vi "SetupProcess.vi"(8 "error in (no error)":errorcluster, 10 "SetupData":string, 11 "ScopeBB in":refnum<class "ScopeBB.lvclass">) -> (0 "error out":errorcluster, 2 "Type":string, 3 "ScopeBB out":refnum<class "ScopeBB.lvclass">)   [LabVIEW 2018, in "ScopeBB.lvclass"]
uses:
  ScopeBB.lvclass
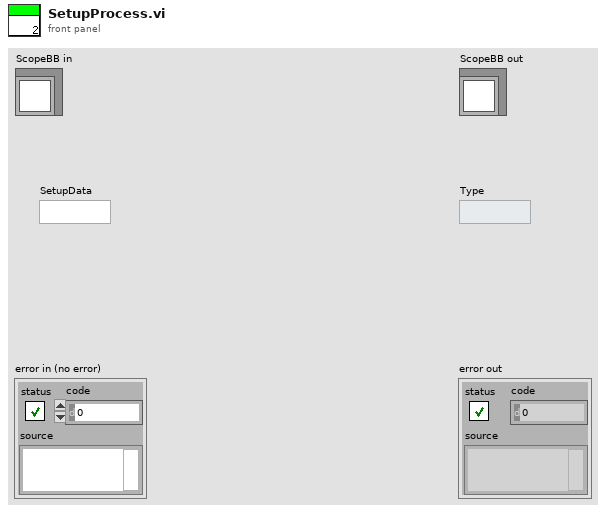
[diagram p1: front panel]
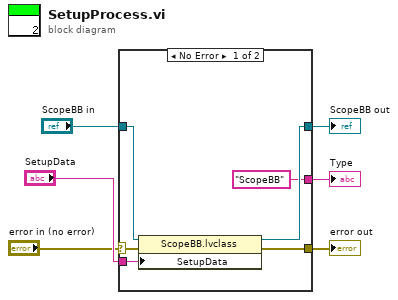
[diagram p0: block diagram]
diagram:
  n1 = case shown="No Error" "error in (no error)" {
    selector: "error in (no error)" -> [w12 w14]
    tunnel: [w11 w14] -> w1
    tunnel: [w9 w13] -> w3
    tunnel: "ScopeBB in" -> [w10 w13]
    tunnel: "SetupData" -> [w8 _]
    tunnel: ["ScopeBB" _] -> w2
    frame No Error {
      n2 = property class="ScopeBB.lvclass"(reference=w10, error in=w12, "SetupData"=w8) -> (reference out=w9:refnum<class "ScopeBB.lvclass">, error out=w11:errorcluster)
    }
    frame Error {
    }
  }
  "error out" <- w1
  "ScopeBB out" <- w3
  "Type" <- w2
